vi "integer_to_7-seg.vi"(10 "Entero":u16 max=15 step=1) -> (2 "7-seg":bool[](array[boolean]))   [LabVIEW 2015]
panel:
  # "Número entero\nentre 0 y 15"
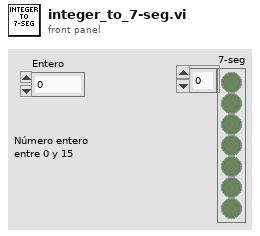
[diagram p1: front panel]
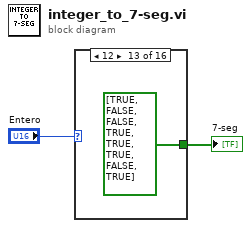
[diagram p0: block diagram]
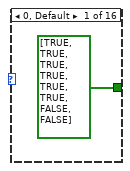
[diagram p2: hidden frame]
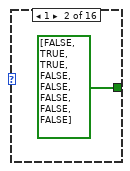
[diagram p3: hidden frame]
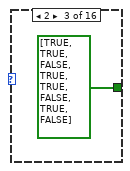
[diagram p4: hidden frame]
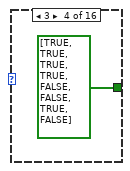
[diagram p5: hidden frame]
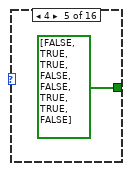
[diagram p6: hidden frame]
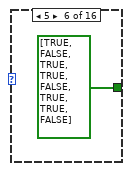
[diagram p7: hidden frame]
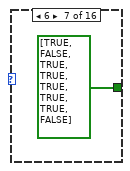
[diagram p8: hidden frame]
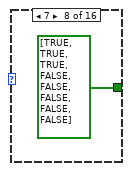
[diagram p9: hidden frame]
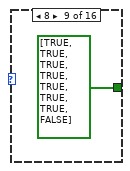
[diagram p10: hidden frame]
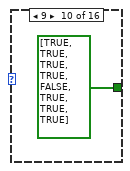
[diagram p11: hidden frame]
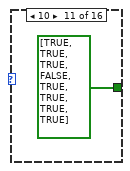
[diagram p12: hidden frame]
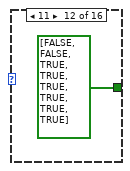
[diagram p13: hidden frame]
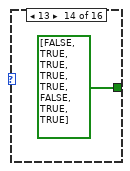
[diagram p14: hidden frame]
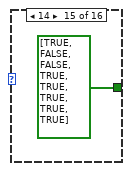
[diagram p15: hidden frame]
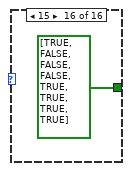
[diagram p16: hidden frame]
diagram:
  n1 = case shown="12" "Entero" {
    tunnel: [bool[] [TRUE, TRUE, TRUE, TRUE, TRUE, TRUE, FALSE, FALSE] bool[] [FALSE, TRUE, TRUE, FALSE, FALSE, FALSE, FALSE, FALSE] bool[] [TRUE, TRUE, FALSE, TRUE, TRUE, FALSE, TRUE, FALSE] bool[] [TRUE, TRUE, TRUE, TRUE, FALSE, FALSE, TRUE, FALSE] bool[] [FALSE, TRUE, TRUE, FALSE, FALSE, TRUE, TRUE, FALSE] bool[] [TRUE, FALSE, TRUE, TRUE, FALSE, TRUE, TRUE, FALSE] bool[] [TRUE, FALSE, TRUE, TRUE, TRUE, TRUE, TRUE, FALSE] bool[] [TRUE, TRUE, TRUE, FALSE, FALSE, FALSE, FALSE, FALSE] bool[] [TRUE, TRUE, TRUE, TRUE, TRUE, TRUE, TRUE, FALSE] bool[] [TRUE, TRUE, TRUE, TRUE, FALSE, TRUE, TRUE, TRUE] bool[] [TRUE, TRUE, TRUE, FALSE, TRUE, TRUE, TRUE, TRUE] bool[] [FALSE, FALSE, TRUE, TRUE, TRUE, TRUE, TRUE, TRUE] bool[] [TRUE, FALSE, FALSE, TRUE, TRUE, TRUE, FALSE, TRUE] bool[] [FALSE, TRUE, TRUE, TRUE, TRUE, FALSE, TRUE, TRUE] bool[] [TRUE, FALSE, FALSE, TRUE, TRUE, TRUE, TRUE, TRUE] bool[] [TRUE, FALSE, FALSE, FALSE, TRUE, TRUE, TRUE, TRUE]] -> w1
    frame 0, Default {
    }
    frame 1 {
    }
    frame 2 {
    }
    frame 3 {
    }
    frame 4 {
    }
    frame 5 {
    }
    frame 6 {
    }
    frame 7 {
    }
    frame 8 {
    }
    frame 9 {
    }
    frame 10 {
    }
    frame 11 {
    }
    frame 12 {
    }
    frame 13 {
    }
    frame 14 {
    }
    frame 15 {
    }
  }
  "7-seg" <- w1
